vi "get_is_complete.vi"(8 "error in (no error)":errorcluster, 11 "Request in":refnum<class "Request.lvclass">) -> (0 "error out":errorcluster, 2 "is_complete":bool, 3 "Request out":refnum<class "Request.lvclass">)   [LabVIEW 2020, in "reqwest.lvlib" / "Request.lvclass"]
uses:
  Request.lvclass
  Request.lvclass/Request.ctl
  lv_reqwest_64.dll
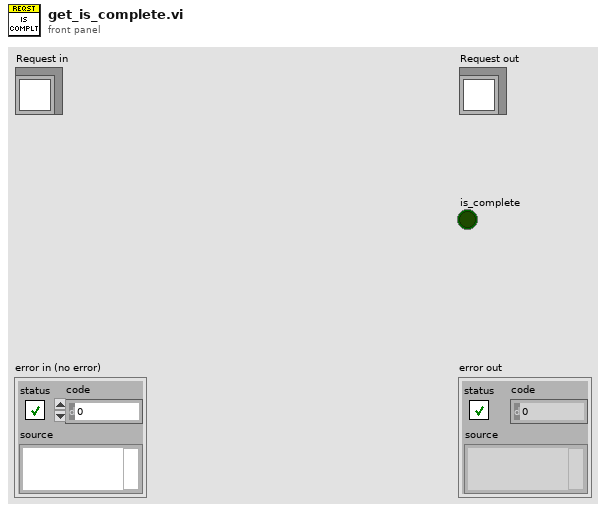
[diagram p1: front panel]
types:
  T1 = typedef "reqwest.lvlib/Request.lvclass/request_id_int.ctl" = u64
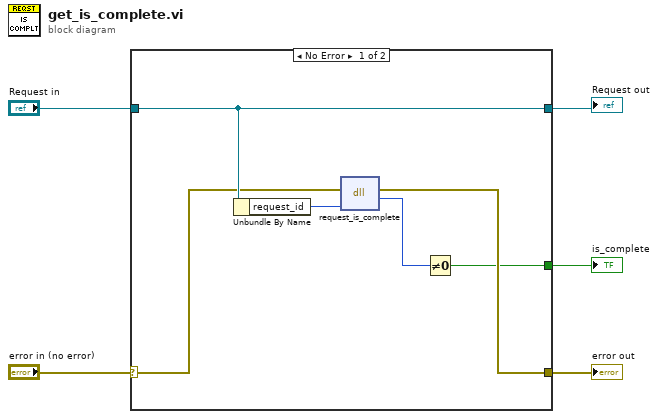
[diagram p0: block diagram]
diagram:
  n1 = case shown="No Error" "error in (no error)" {
    selector: "error in (no error)" -> [w9 w12]
    tunnel: "Request in" -> [w10 w13]
    tunnel: [w7 _] -> w3
    tunnel: [w11 w12] -> w1
    tunnel: [w10 w13] -> w2
    frame No Error {
      n2 = Unbundle By Name(w10) -> ("request_id"=w8:T1)
      n3 = dll-call lib="C:/Projects/reqwest-rs-labview/lv_src/lv_reqwest_*.*" fn="request_is_complete"(error in=w9, "request_id"=w8) -> (error out=w11:errorcluster, "is_complete"=w6:u8)  [unwired: 3 in, 1 out]
      n4 = Not Equal To 0?(x=w6) -> (x != 0?=w7:bool)
    }
    frame Error {
    }
  }
  "error out" <- w1
  "is_complete" <- w3
  "Request out" <- w2
